vi "Initialize Tree.vi"(7 "path":path, 8 "error in":errorcluster, 10 "reference":refnum<vi>, 11 "tdms file":refnum<k34>) -> (0 "error out":errorcluster, 2 "Tree Ref out":refnum<vi>, 3 "tdms file out":refnum<k34>)   [LabVIEW 2017, in "Report Viewer.lvlib"]
uses:
  Report Viewer.lvlib
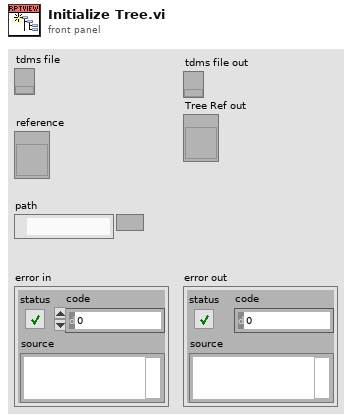
[diagram p1: front panel]
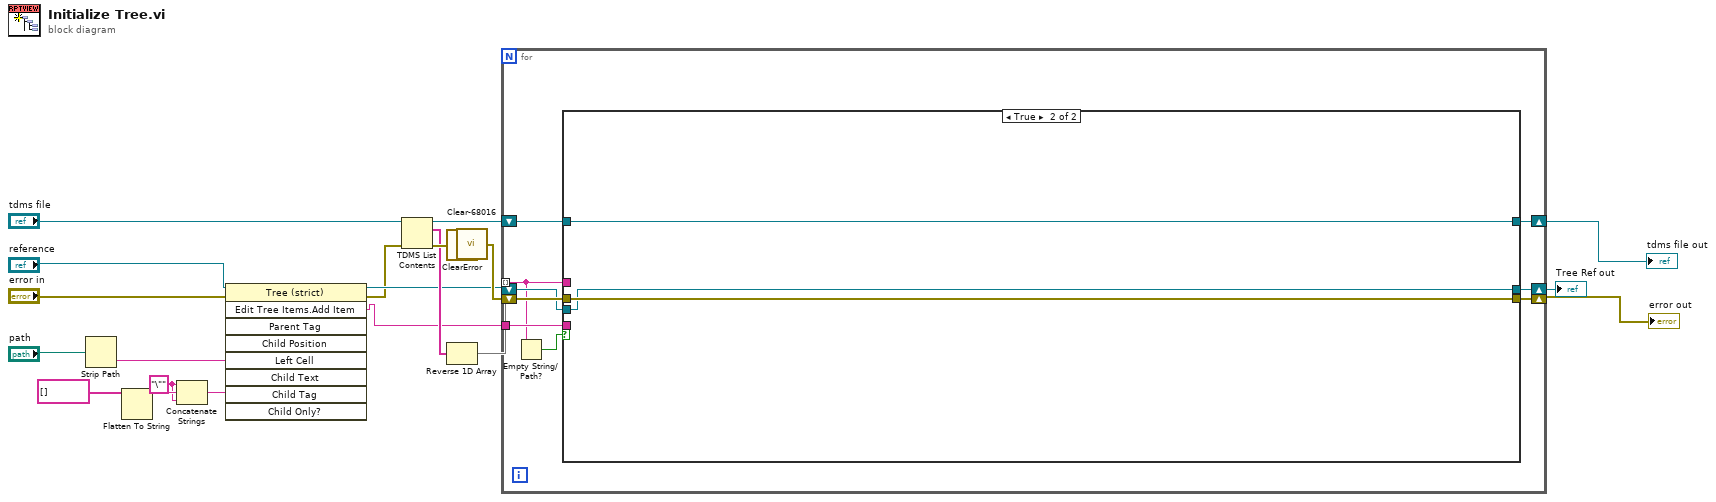
[diagram p0: block diagram]
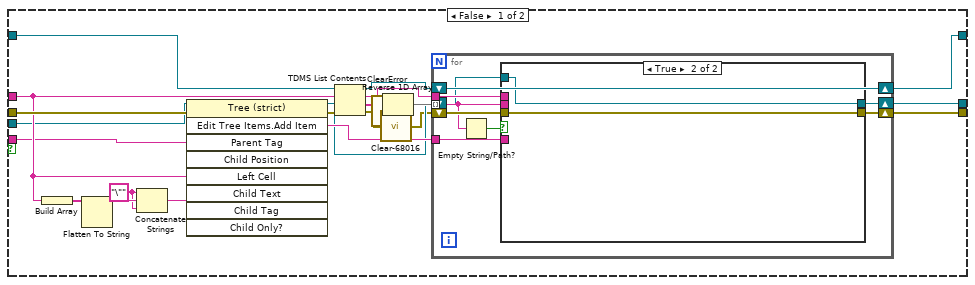
[diagram p2: hidden frame]
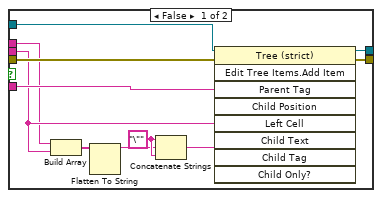
[diagram p3: hidden frame]
diagram:
  w13 = "\"" ("string")
  n1 = Strip Path(path="path") -> (name=w12:string)  [unwired: 1 out]
  n2 = Flatten To String(anything=string[] [] ("appended array")) -> (data string=w14:string)  [unwired: 3 in, 2 out]
  n3 = Concatenate Strings(w13, w14, w13) -> (w16:string)
  n4 = invoke on="Invoke Node" class="Tree (strict)" method="Edit Tree Items.Add Item"(reference="reference", error in="error in", "Left Cell"=w12, "Child Tag"=w16) -> (reference out=w11:refnum<vi>, error out=w10:errorcluster, "Edit Tree Items:Add Item"=w17:string)  [unwired: 5 in, 6 out]
  n5 = TDMS List Contents(4:w10, 7:"tdms file") -> (0:w21:errorcluster, 2:w18:string[], 3:w9:refnum<k34>)  [unwired: 1 in, 1 out]
  n6 = call <vilib>:"ClearError.vi"("error in (no error)"=w21) -> ("error out"=w19:errorcluster)
  n7 = Reverse 1D Array(array=w18) -> (reversed array=w8:string[])
  n8 = call <vilib>:"Clear-68016.vi"("error in (no error)"=w19) -> ("error out"=w20:errorcluster)
  n9 = for {
    tunnel: w8 -> [w24] mode=indexing
    shift-right: [w27] -> w2
    shift-left: w9 -> [w29]
    shift-right: [w28] -> w7
    shift-left: w20 -> [w30]
    tunnel: w17 -> [w25]
    shift-right: [w22] -> w1
    shift-left: w11 -> [w26]
    n10 = Empty String/Path?(string/path=w24) -> (empty?=w23:bool)
    n11 = case shown="True" w23 {
      tunnel: w30 -> [w52 w76]
      tunnel: w29 -> [w50 w77]
      tunnel: [w49 w76] -> w28
      tunnel: [w47 w77] -> w27
      tunnel: w24 -> [w45 _]
      tunnel: w26 -> [w38 w75]
      tunnel: w25 -> [w36 _]
      tunnel: [w31 w75] -> w22
      frame False {
        w39 = "\"" ("string")
        n12 = Build Array(w45) -> (w44:string[])
        n13 = Flatten To String(anything=w44) -> (data string=w41:string)  [unwired: 3 in, 2 out]
        n14 = Concatenate Strings(w39, w41, w39) -> (w40:string)
        n15 = invoke on="Invoke Node" class="Tree (strict)" method="Edit Tree Items.Add Item"(reference=w38, error in=w52, "Parent Tag"=w36, "Left Cell"=w45, "Child Tag"=w40) -> (reference out=w37:refnum<vi>, error out=w51:errorcluster, "Edit Tree Items:Add Item"=w46:string)  [unwired: 4 in, 6 out]
        n16 = TDMS List Contents(4:w51, 6:w45, 7:w50) -> (0:w32:errorcluster, 1:w35:string[], 2:w43:string, 3:w48:refnum<k34>)
        n17 = call <vilib>:"ClearError.vi"("error in (no error)"=w32) -> ("error out"=w34:errorcluster)
        n18 = call <vilib>:"Clear-68016.vi"("error in (no error)"=w34) -> ("error out"=w33:errorcluster)
        n19 = Reverse 1D Array(array=w35) -> (reversed array=w42:string[])
        n20 = for {
          tunnel: w42 -> [w55] mode=indexing
          shift-right: [w59] -> w47
          shift-left: w48 -> [w59]
          shift-right: [w60] -> w49
          shift-left: w33 -> [w61]
          tunnel: w46 -> [w58]
          tunnel: w43 -> [w57]
          shift-right: [w53] -> w31
          shift-left: w37 -> [w54]
          n21 = Empty String/Path?(string/path=w55) -> (empty?=w56:bool)
          n22 = case shown="True" w56 {
            tunnel: w61 -> [w72 w74]
            tunnel: [w71 w74] -> w60
            tunnel: w58 -> [w70 _]
            tunnel: w55 -> [w68 _]
            tunnel: w57 -> [w67 _]
            tunnel: w54 -> [w63 w73]
            tunnel: [w62 w73] -> w53
            frame False {
              w66 = "\"" ("string")
              n23 = Build Array(w67, w68) -> (w69:string[])
              n24 = Flatten To String(anything=w69) -> (data string=w64:string)  [unwired: 3 in, 2 out]
              n25 = Concatenate Strings(w66, w64, w66) -> (w65:string)
              n26 = invoke on="Invoke Node" class="Tree (strict)" method="Edit Tree Items.Add Item"(reference=w63, error in=w72, "Parent Tag"=w70, "Left Cell"=w68, "Child Tag"=w65) -> (reference out=w62:refnum<vi>, error out=w71:errorcluster)  [unwired: 4 in, 7 out]
            }
            frame True {
            }
          }
        }
      }
      frame True {
      }
    }
  }
  "error out" <- w7
  "tdms file out" <- w2
  "Tree Ref out" <- w1
